vi "QVA_TrimSpacesAndBrackets.vi"(2 "String":string) -> (16 "TrimmedString":string)   [LabVIEW 2016]
doc: "Entfernt Klammern und leere Zeichen am Anfang und Ende des Strings\n\nsige / 3.12.13"
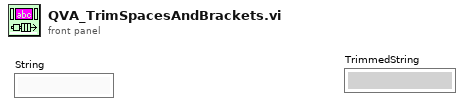
[diagram p1: front panel]
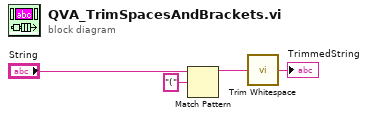
[diagram p0: block diagram]
diagram:
  n1 = Match Pattern(string="String", regular expression="(") -> (before substring=w4:string)  [unwired: 1 in, 3 out]
  n2 = call <vilib>:"Trim Whitespace.vi"("string"=w4) -> ("trimmed string"=→"TrimmedString":string)  [unwired: 1 in]
